vi "Send Log Delimiter Message.vi"(8 "error in (no error)":errorcluster, 10 "Log Delimiter":string, 11 "Generic Controller in":refnum<class "Generic Plugin.lvclass">) -> (0 "error out":errorcluster, 3 "Generic Controller out":refnum<class "Generic Plugin.lvclass">)   [LabVIEW 2020, in "RxnRover.lvlib" / "Generic Plugin.lvclass"]
uses:
  Generic Plugin.lvclass
  Generic Plugin.lvclass/Generic Plugin.ctl
  <userlib>/RxnRover/DynamicReentrant/Dynamic Reentrant.lvlib
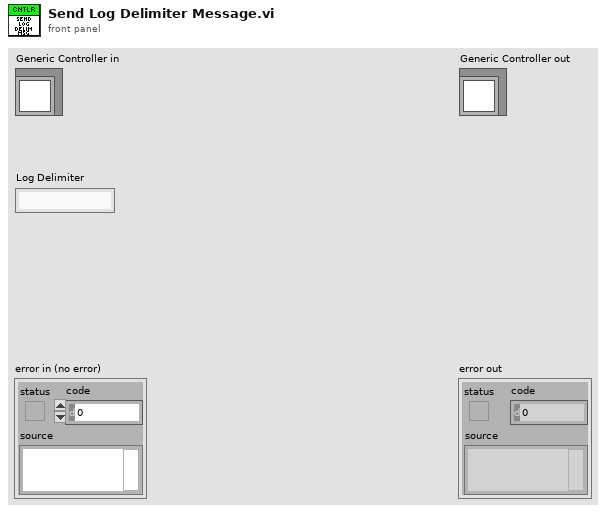
[diagram p1: front panel]
types:
  T1 = typedef "Dynamic Reentrant.lvlib/Message.ctl" = cluster{"Source":string, "Destination":string, "Time Stamp":timestamp, "Command":string, "Data":variant}
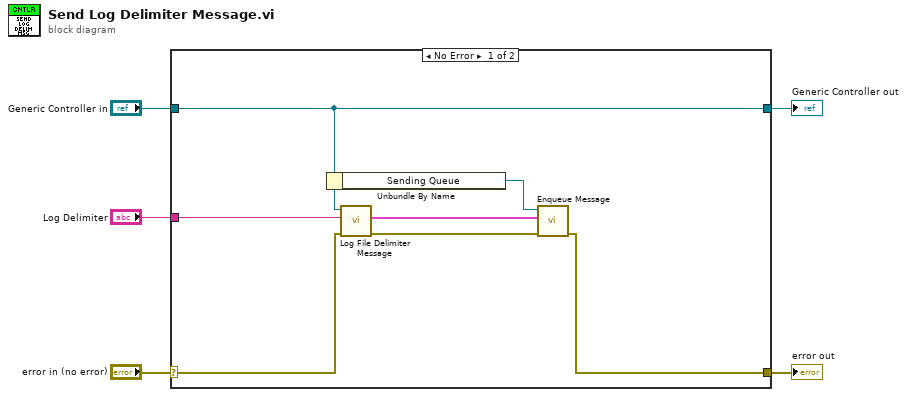
[diagram p0: block diagram]
diagram:
  n1 = case shown="No Error" "error in (no error)" {
    selector: "error in (no error)" -> [w12 w14]
    tunnel: [w7 w14] -> w4
    tunnel: [w11 w13] -> w2
    tunnel: "Generic Controller in" -> [w11 w13]
    tunnel: "Log Delimiter" -> [w6 _]
    frame No Error {
      n2 = Unbundle By Name(w11) -> ("Sending Queue"=w10:refnum<queue>)
      n3 = call-dynamic "Log File Delimiter Message.vi"("error in (no error)"=w12, "Log Delimiter"=w6, "Generic Controller in"=w11) -> ("error out"=w8:errorcluster, "Log File Delimiter Message"=w9:T1)  [unwired: 6 in, 1 out]
      n4 = call <userlib>:"Enqueue Message.vi"("error in (no error)"=w8, "Message"=w9, "Listening Queue"=w10) -> ("error out"=w7:errorcluster)  [unwired: 7 in, 1 out]
    }
    frame Error {
    }
  }
  "error out" <- w4
  "Generic Controller out" <- w2
